vi "CSDB_Config.delete instances.vi"(2 "Names":string[](array[string]), 5 "error in (no error)":errorcluster) -> (19 "error out":errorcluster)   [LabVIEW 2014, in "CSDB_Config.lvlib"]
doc: "Deletes instances together with their data from the database."
uses:
  CSDB_Config.lvlib
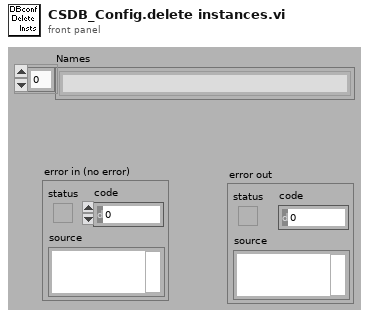
[diagram p1: front panel]
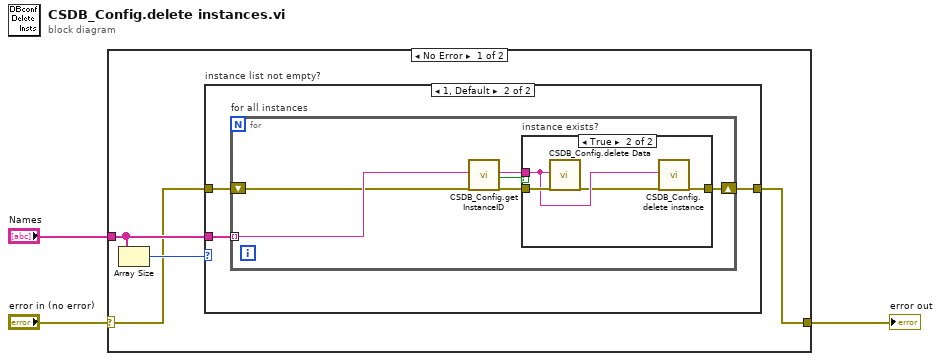
[diagram p0: block diagram]
diagram:
  n1 = case shown="No Error" "error in (no error)" {
    selector: "error in (no error)" -> [w5 w23]
    tunnel: "Names" -> [w6 _]
    tunnel: [w4 w23] -> w2
    frame No Error {
      n2 = Array Size(array=w6) -> (size(s)=w7:i32)
      n3 = case "instance list not empty?" shown="1, Default" w7 {
        tunnel: w6 -> [_ w11]
        tunnel: w5 -> [w8 w10]
        tunnel: [w8 w9] -> w4
        frame 0 {
        }
        frame 1, Default {
          n4 = for "for all instances" {
            tunnel: w11 -> [w15] mode=indexing
            shift-right: [w12] -> w9
            shift-left: w10 -> [w13]
            n5 = call "CSDB_Config.get InstanceID.vi"("InstanceName"=w15, "error in (no error)"=w13) -> ("InstanceID"=w17:string, "entry exists?"=w14:bool, "error out"=w16:errorcluster)  [unwired: 15 in]
            n6 = case "instance exists?" shown="True" w14 {
              tunnel: w17 -> [_ w21]
              tunnel: w16 -> [w18 w22]
              tunnel: [w18 w19] -> w12
              frame False {
              }
              frame True {
                n7 = call "CSDB_Config.delete Data.vi"("InstanceID"=w21, "error in (no error)"=w22) -> ("error out"=w20:errorcluster)  [unwired: 17 in]
                n8 = call "CSDB_Config.delete instance.vi"("InstanceID"=w21, "error in (no error)"=w20) -> ("error out"=w19:errorcluster)  [unwired: 17 in]
              }
            }
          }
        }
      }
    }
    frame Error {
    }
  }
  "error out" <- w2
